vi "Set Time.vi"(8 "error IO":errorcluster, 10 "Time":string, 11 "VISA resource name":refnum<visa-resource-name>) -> (0 "error Out":errorcluster, 3 "VISA resource Out":refnum<visa-resource-name>)   [LabVIEW 2012, in "Associated Research 78XX Series.lvlib"]
uses:
  <instrlib>/Associated Research 78XX Series/Associated Research 78XX Series.lvlib
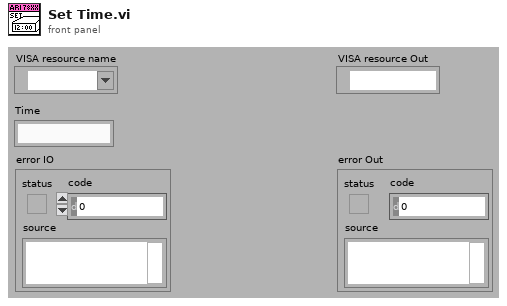
[diagram p1: front panel]
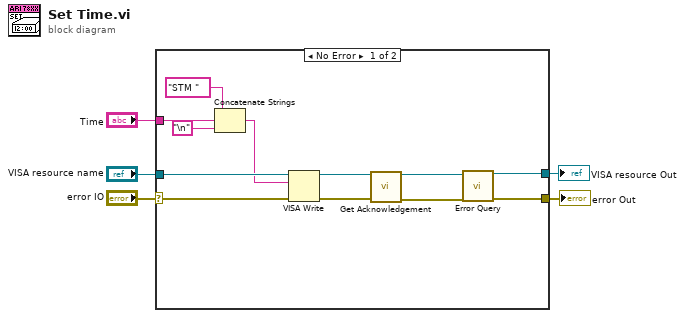
[diagram p0: block diagram]
diagram:
  n1 = case shown="No Error" "error IO" {
    selector: "error IO" -> [w17 w19]
    tunnel: [w14 w19] -> w2
    tunnel: [w15 w18] -> w3
    tunnel: "VISA resource name" -> [w16 w18]
    tunnel: "Time" -> [w10 _]
    frame No Error {
      n2 = Concatenate Strings("STM " ("Command to Send (empty)"), w10, "\n") -> (w11:string)
      n3 = VISA Write(VISA resource name=w16, write buffer=w11, error in (no error)=w17) -> (VISA resource name out=w7:refnum<visa-resource-name>, error out=w6:errorcluster)  [unwired: 1 out]
      n4 = call <instrlib>:"Get Acknowledgement.vi"("VISA resource name"=w7, "error in (no error)"=w6) -> ("VISA resource name out"=w9:refnum<visa-resource-name>, "error out"=w8:errorcluster)  [unwired: 12 in]
      n5 = call <instrlib>:"Error Query.vi"("VISA resource name"=w9, "error in (no error)"=w8) -> ("VISA resource name out"=w15:refnum<visa-resource-name>, "error out"=w14:errorcluster)  [unwired: 10 in, 2 out]
    }
    frame Error {
    }
  }
  "VISA resource Out" <- w3
  "error Out" <- w2
